vi "Default Responses.vi"() -> (2 "Default Failed Response":refnum<class "Response.lvclass">, 3 "Default Success Response":refnum<class "Response.lvclass">)   [LabVIEW 2020, in "OAuth2.lvlib"]
doc: "Defines the default responses that are returned to the user upon completing an authorization flow either successfully or from a failed request. This VI is used to generate the class values that are stored as default values for the optional inputs in the Do Auth VI."
uses:
  OAuth2.lvlib
  <vilib>/IlluminatedG/IG HTTP Utils/HTTP Utils/Response/Response.lvclass
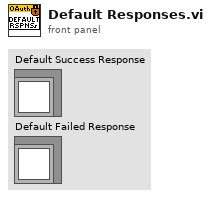
[diagram p1: front panel]
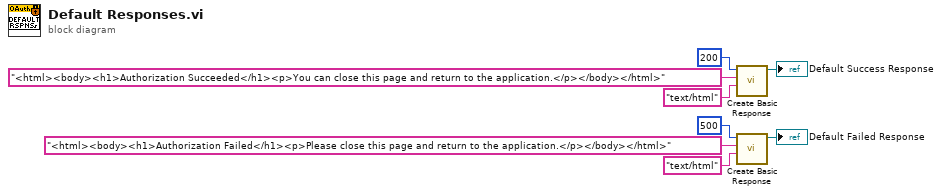
[diagram p0: block diagram]
diagram:
  n1 = call <vilib>:"Create Basic Response.vi"("Content-Type (text/plain)"="text/html", "Payload"="<html><body><h1>Authorization Succeeded</h1><p>You can close this page and return to the application.</p></body></html>" ("Success Response (Default)"), "Status Code"=u16 200) -> ("Response out"=→"Default Success Response":refnum<class "Response.lvclass">)  [unwired: 7 in, 1 out]
  n2 = call <vilib>:"Create Basic Response.vi"("Content-Type (text/plain)"="text/html", "Payload"="<html><body><h1>Authorization Failed</h1><p>Please close this page and return to the application.</p></body></html>" ("Success Response (Default)"), "Status Code"=u16 500) -> ("Response out"=→"Default Failed Response":refnum<class "Response.lvclass">)  [unwired: 7 in, 1 out]
